vi "Comm_read 1d cdb.vi"(8 "error in (no error)":errorcluster, 10 "timeout in ms (-1)":i32=-1, 11 "WPL Comm (1D CDB) in":refnum<class "WPL Comm (1D CDB).lvclass">) -> (0 "error out":errorcluster, 1 "Properties":T1, 2 "Data":cdb[](array[numeric]), 4 "timed out?":bool)   [LabVIEW 2020, in "Internal Comm Classes.lvlib" / "WPL Comm (1D CDB).lvclass"]
uses:
  WPL Comm (1D CDB).lvclass
  Waveform properties.ctl
  Custom Device API/Waveform Data Reference.ctl
  WPL Comm (1D CDB).lvclass/WPL Comm (1D CDB).ctl
  WPL Comm.lvclass
  NI_VS Custom Device Waveform API.lvlib
  Custom Device API/Custom Device API.lvlib
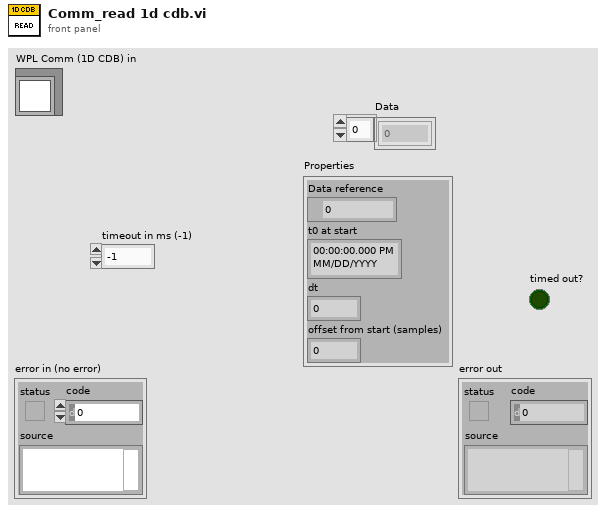
[diagram p1: front panel]
types:
  T1 = typedef "NI_VS Custom Device Waveform API.lvlib/Waveform properties.ctl" = cluster{"Data reference":T2, "t0 at start":timestamp, "dt":dbl, "offset from start (samples)":u64}
  T2 = typedef "Custom Device API.lvlib/Waveform Data Reference.ctl" = i32
  T3 = typedef "Internal Comm Classes.lvlib/WPL Comm (1D CDB).lvclass/Waveform 1d cdb read queue.ctl" = refnum<queue>
  T4 = typedef "Internal Comm Classes.lvlib/WPL Comm (1D CDB).lvclass/Waveform 1d cdb read cluster.ctl" = cluster{"Waveform Properties":T1, "Data":cdb[]}
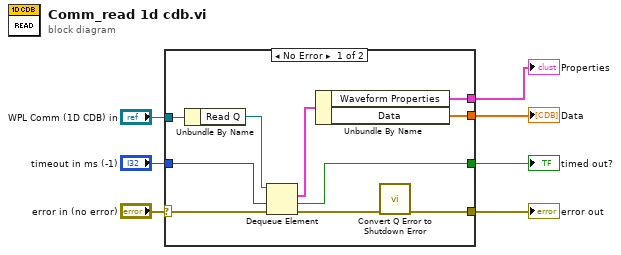
[diagram p0: block diagram]
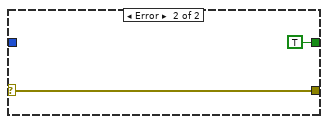
[diagram p2: hidden frame]
diagram:
  n1 = case shown="No Error" "error in (no error)" {
    selector: "error in (no error)" -> [w8 w19]
    tunnel: "timeout in ms (-1)" -> [w17 _]
    tunnel: "WPL Comm (1D CDB) in" -> [w16 _]
    tunnel: [w13 _] -> w5
    tunnel: [w12 _] -> w4
    tunnel: [w10 w19] -> w3
    tunnel: [w9 TRUE ("timed out?")] -> w2
    frame No Error {
      n2 = Unbundle By Name(w16) -> ("Read Q"=w15:T3)
      n3 = Dequeue Element(queue=w15, timeout in ms (-1)=w17, error in (no error)=w8) -> (element=w14:T4, timed out?=w9:bool, error out=w11:errorcluster)  [unwired: 1 out]
      n4 = Unbundle By Name(w14) -> ("Waveform Properties"=w13:T1, "Data"=w12:cdb[])
      n5 = call "Convert Q Error to Shutdown Error.vi"("error in (no error)"=w11) -> ("error out"=w10:errorcluster)  [unwired: 10 in]
    }
    frame Error {
    }
  }
  "error out" <- w3
  "Properties" <- w5
  "Data" <- w4
  "timed out?" <- w2
